vi "Read Environment Variable.vi"(8 "error in":errorcluster, 11 "name":string) -> (0 "error out":errorcluster, 3 "value":string)   [LabVIEW 2021, in "NI Discovery V1 Client.lvlib"]
uses:
  NI Discovery V1 Client.lvlib
  <vilib>/Utility/error.llb/Trim Whitespace One-Sided.vi
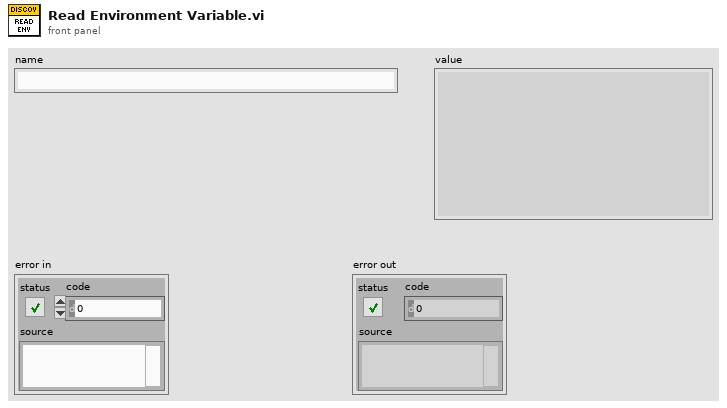
[diagram p1: front panel]
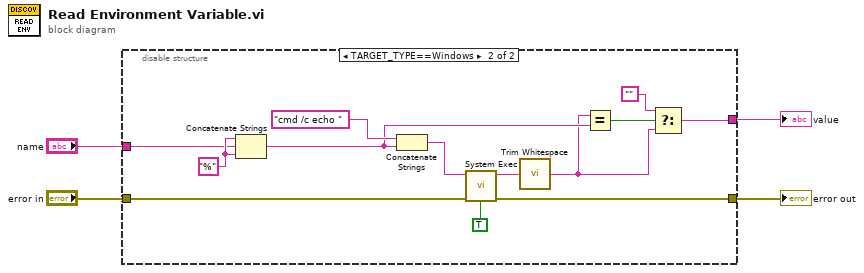
[diagram p0: block diagram]
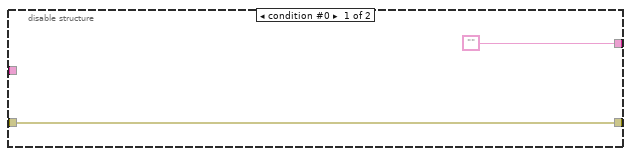
[diagram p2: hidden frame]
diagram:
  n1 = disable-structure shown="TARGET_TYPE==Windows" {
    disable-tunnel: "error in" -> [w5 w16]
    disable-tunnel: [w5 w15] -> w3
    disable-tunnel: ["" w8] -> w1
    disable-tunnel: "name" -> [_ w13]
    frame condition #0 {
    }
    frame condition #1 (active) {
      w14 = "%" ("string")
      n2 = Concatenate Strings(w14, w13, w14) -> (w12:string)
      n3 = Concatenate Strings("cmd /c echo " ("string"), w12) -> (w19:string)
      n4 = call <vilib>:"System Exec.vi"("run minimized? (F)"=TRUE, "error in (no error)"=w16, "command line"=w19) -> ("error out"=w15:errorcluster, "standard output"=w9:string)  [unwired: 5 in, 2 out]
      n5 = call <vilib>:"Trim Whitespace.vi"("string"=w9) -> ("trimmed string"=w7:string)  [unwired: 1 in]
      n6 = Equal?(x=w7, y=w12) -> (x = y?=w11:bool)
      n7 = Select(t="", s=w11, f=w7) -> (s? t:f=w8:string)
    }
  }
  "error out" <- w3
  "value" <- w1
